vi "Fix Paired Channels.vi"(0 "Paired E2E configuration in":refnum<class "E2E Tag Exchange configuration.lvclass">, 5 "Paired engine configuration in":refnum<class "engine configuration.lvclass">, 7 "E2E configuration in":refnum<class "E2E Tag Exchange configuration.lvclass">, 9 "engine configuration in":refnum<class "engine configuration.lvclass">, 11 "error in (no error)":errorcluster) -> (4 "Paired E2E configuration out":refnum<class "E2E Tag Exchange configuration.lvclass">, 6 "Paired engine configuration out":refnum<class "engine configuration.lvclass">, 8 "E2E configuration out":refnum<class "E2E Tag Exchange configuration.lvclass">, 10 "engine configuration out":refnum<class "engine configuration.lvclass">, 15 "error out":errorcluster)   [LabVIEW 2015, in "E2E Tag Exchange editor node.lvclass"]
uses:
  E2E Tag Exchange editor node.lvclass
  module/configuration/E2E Tag Exchange configuration.lvclass
  <vilib>/NI/Module Execution Interface/Engine Configuration/engine configuration.lvclass
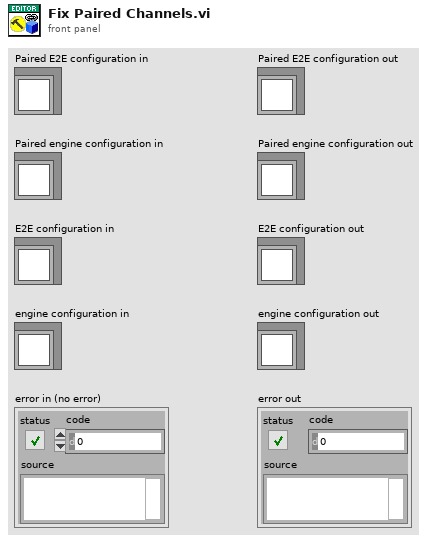
[diagram p1: front panel]
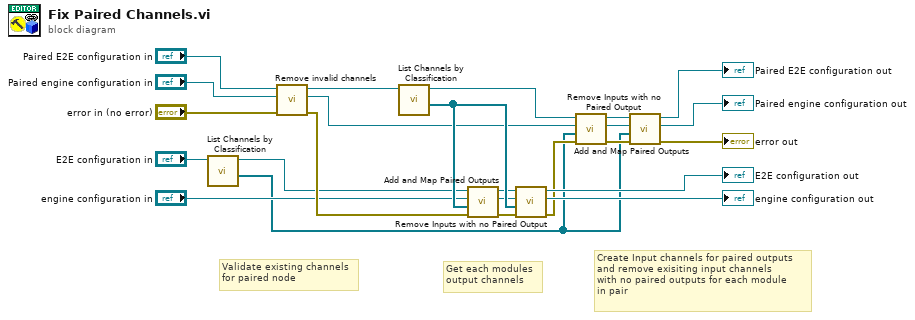
[diagram p0: block diagram]
diagram:
  # "Get each modules\noutput channels"
  # "Create Input channels for paired outputs\nand remove exisiting input channels\nwith no paired outputs for each module\nin pair"
  # "Validate existing channels\nfor paired node"
  n1 = call "List Channels by Classification.vi"("E2E configuration in"="E2E configuration in") -> ("Output Channels"=w10:refnum<class "TBM channel.lvclass">[], "E2E configuration out"=w7:refnum<class "E2E Tag Exchange configuration.lvclass">)  [unwired: 8 in, 1 out]
  n2 = call "Remove invalid channels.vi"("error in (no error)"="error in (no error)", "engine configuration in"="Paired engine configuration in", "E2E configuration in"="Paired E2E configuration in") -> ("error out"=w16:errorcluster, "engine configuration out"=w8:refnum<class "engine configuration.lvclass">, "E2E configuration out"=w23:refnum<class "E2E Tag Exchange configuration.lvclass">)  [unwired: 6 in]
  n3 = call "List Channels by Classification.vi"("E2E configuration in"=w23) -> ("Output Channels"=w15:refnum<class "TBM channel.lvclass">[], "E2E configuration out"=w6:refnum<class "E2E Tag Exchange configuration.lvclass">)  [unwired: 8 in, 1 out]
  n4 = call "Add and Map Paired Outputs.vi"("error in (no error)"=w16, "Paired Module Output Channels"=w15, "engine configuration in"="engine configuration in", "E2E configuration in"=w7) -> ("error out"=w17:errorcluster, "engine configuration out"=w14:refnum<class "engine configuration.lvclass">, "E2E configuration out"=w13:refnum<class "E2E Tag Exchange configuration.lvclass">)  [unwired: 5 in]
  n5 = call "Remove Inputs with no Paired Output.vi"("error in (no error)"=w17, "Paired Module Output Channels"=w15, "engine configuration in"=w14, "E2E configuration in"=w13) -> ("error out"=w18:errorcluster, "engine configuration out"=→"engine configuration out":refnum<class "engine configuration.lvclass">, "E2E configuration out"=→"E2E configuration out":refnum<class "E2E Tag Exchange configuration.lvclass">)  [unwired: 5 in]
  n6 = call "Add and Map Paired Outputs.vi"("error in (no error)"=w18, "Paired Module Output Channels"=w10, "engine configuration in"=w8, "E2E configuration in"=w6) -> ("error out"=w19:errorcluster, "engine configuration out"=w11:refnum<class "engine configuration.lvclass">, "E2E configuration out"=w9:refnum<class "E2E Tag Exchange configuration.lvclass">)  [unwired: 5 in]
  n7 = call "Remove Inputs with no Paired Output.vi"("error in (no error)"=w19, "Paired Module Output Channels"=w10, "engine configuration in"=w11, "E2E configuration in"=w9) -> ("error out"=→"error out":errorcluster, "engine configuration out"=→"Paired engine configuration out":refnum<class "engine configuration.lvclass">, "E2E configuration out"=→"Paired E2E configuration out":refnum<class "E2E Tag Exchange configuration.lvclass">)  [unwired: 5 in]
